vi "nirviErrorMergeTemplate.vi"(1 "error array in":errorcluster[](array[cluster])) -> (0 "error out":errorcluster)   [LabVIEW 2017]
doc: "Merges error I/O clusters from different functions."
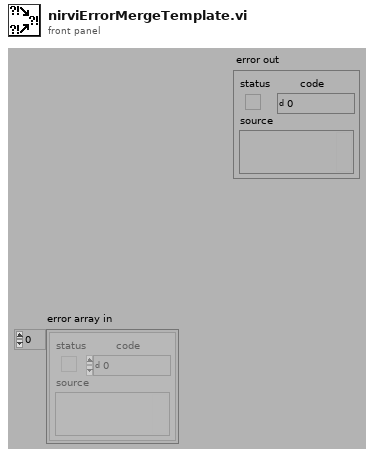
[diagram p1: front panel]
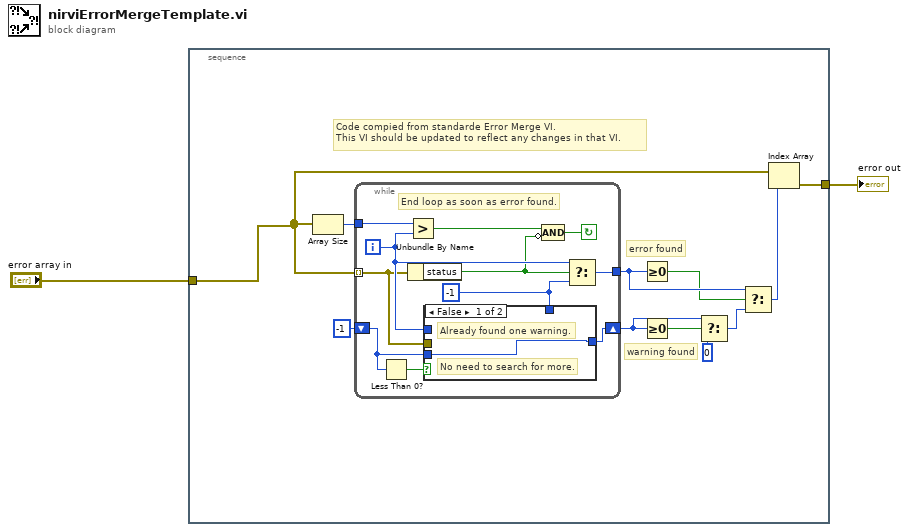
[diagram p0: block diagram]
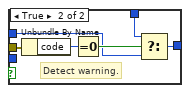
[diagram p2: hidden frame]
diagram:
  n1 = stacked-sequence {
    tunnel: [w13] -> w2
    tunnel: "error array in" -> [w12]
    frame #0 {
      # "Code compied from standarde Error Merge VI.\nThis VI should be updated to reflect any changes in that VI."
      # "warning found"
      # "error found"
      n2 = Array Size(array=w12) -> (size(s)=w11:i32)
      n3 = while {
        tunnel: w11 -> [w24]
        tunnel: [w21] -> w10
        tunnel: w12 -> [w17] mode=indexing
        shift-right: [w15] -> w8
        shift-left: -1 -> [w14]
        i -> [w19]
        stop <- w22 continue-if-true
        w20 = -1
        # "End loop as soon as error found."
        n4 = Less Than 0?(x=w14) -> (x < 0?=w16:bool)
        n5 = Greater?(x=w24, y=w19) -> (0:w23:bool)
        n6 = Unbundle By Name(w17) -> ("status"=w18:bool)
        n7 = case shown="False" w16 {
          tunnel: w20 -> [_ w29]
          tunnel: w19 -> [_ w28]
          tunnel: w17 -> [_ w27]
          tunnel: [w25 w26] -> w15
          tunnel: w14 -> [w25 _]
          frame False {
            # "No need to search for more."
            # "Already found one warning."
          }
          frame True {
            # "Detect warning."
            n8 = Unbundle By Name(w27) -> ("code"=w31:i32)
            n9 = Equal To 0?(x=w31) -> (x = 0?=w30:bool)
            n10 = Select(t=w29, s=w30, f=w28) -> (s? t:f=w26:i32)
          }
        }
        n11 = Compound Arithmetic op=AND(w23, invert w18) -> (w22:bool)
        n12 = Select(t=w19, s=w18, f=w20) -> (s? t:f=w21:i32)
      }
      n13 = Greater Or Equal To 0?(x=w10) -> (x >= 0?=w9:bool)
      n14 = Greater Or Equal To 0?(x=w8) -> (x >= 0?=w7:bool)
      n15 = Select(t=w8, s=w7, f=0) -> (s? t:f=w5:i32)
      n16 = Select(t=w10, s=w9, f=w5) -> (s? t:f=w4:i32)
      n17 = Index Array(array=w12, index=w4) -> (element=w13:errorcluster)
    }
  }
  "error out" <- w2
